vi "FilterNetworkStreamErrors.vi"(8 "error in (no error)":errorcluster) -> (0 "error out":errorcluster, 2 "NetStream Error?":bool)   [LabVIEW 2023, in "NetworkConnection.lvclass"]
doc: "Checks for specific Network Streams erros and clears them if found.\n\nJKI Network Streams Connection 1.1.1.15\nJavier Ruiz - JKI\nCopyright (c) 2020, JKI\n\nThis library is provided \"AS IS\" ,WITHOUT WARRANTIES OR CONDITIONS OF ANY KIND, either express or implied."
uses:
  NetworkConnection.lvclass
  NetworkConnection.lvclass/NetworkConnection.ctl
panel:
  # "Copyright © 2020 JKI All rights reserved.\n\nAuthor: Javier Ruiz <javier.ruiz@jki.net>\n\nThis library is provided \"AS IS\" ,WITHOUT WARRANTIES OR \nCONDITIONS OF ANY KIND, either expressed or implied.\n\nJKI -- jki.net"
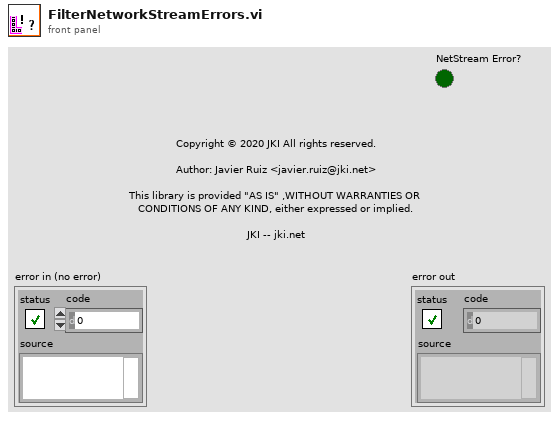
[diagram p1: front panel]
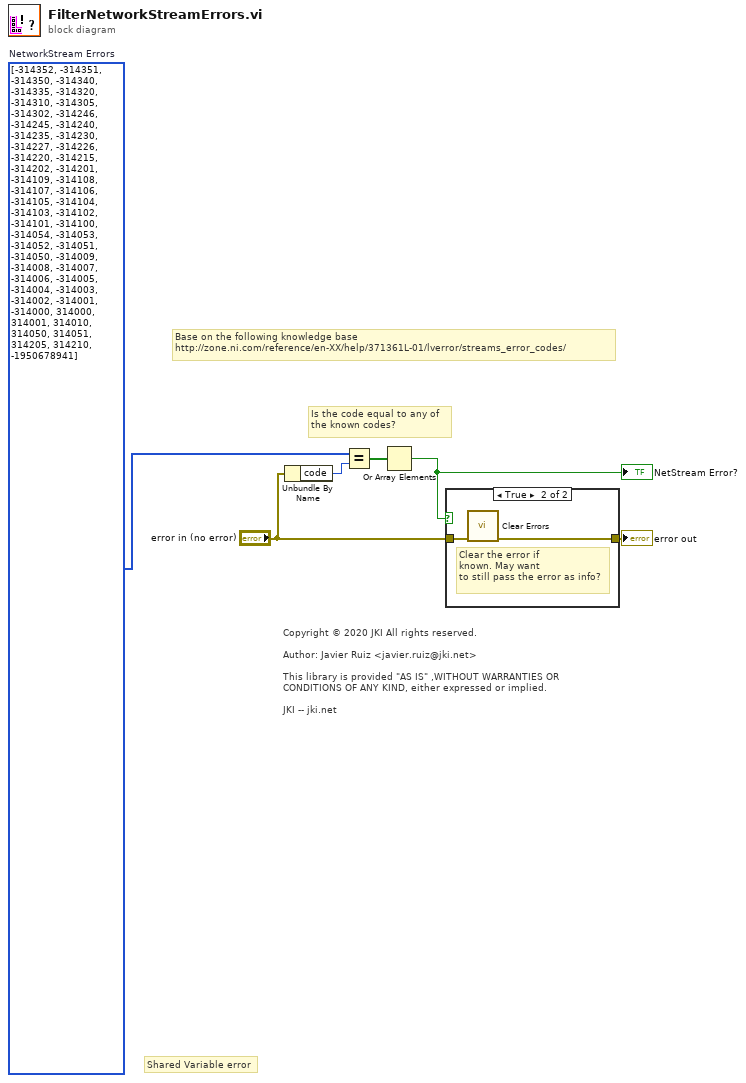
[diagram p0: block diagram]
diagram:
  w3 = i32[] [-314352, -314351, -314350, -314340, -314335, -314320, -314310, -314305, -314302, -314246, -314245, -314240, -314235, -314230, -314227, -314226, -314220, -314215, -314202, -314201, -314109, -314108, -314107, -314106, -314105, -314104, -314103, -314102, -314101, -314100, -314054, -314053, -314052, -314051, -314050, -314009, -314008, -314007, -314006, -314005, -314004, -314003, -314002, -314001, -314000, 314000, 314001, 314010, 314050, 314051, 314205, 314210, -1950678941]  # NetworkStream Errors
  # "Is the code equal to any of\nthe known codes?"
  # "Shared Variable error"
  # "Base on the following knowledge base\nhttp://zone.ni.com/reference/en-XX/help/371361L-01/lverror/streams_error_codes/"
  # "Copyright © 2020 JKI All rights reserved.\n\nAuthor: Javier Ruiz <javier.ruiz@jki.net>\n\nThis library is provided \"AS IS\" ,WITHOUT WARRANTIES OR \nCONDITIONS OF ANY KIND, either expressed or implied.\n\nJKI -- jki.net"
  n1 = Unbundle By Name("error in (no error)") -> ("code"=w4:i32)
  n2 = Equal?(x=w3, y=w4) -> (x = y?=w2:bool[])
  n3 = Or Array Elements(Boolean array=w2) -> (logical OR=w1:bool)
  "NetStream Error?" <- w1
  n4 = case shown="True" w1 {
    tunnel: "error in (no error)" -> [w7 w9]
    tunnel: [w7 w8] -> w5
    frame False {
    }
    frame True {
      # "Clear the error if\nknown. May want\nto still pass the error as info?"
      n5 = call <vilib>:"Clear Errors.vi"("error in (no error)"=w9) -> ("error out"=w8:errorcluster)  [unwired: 5 in, 1 out]
    }
  }
  "error out" <- w5
